vi "Fast Item Remove FuncGlobal.vi"(5 "Action":enum16{"Open or Add", "Close Ref"}(ring), 8 "error in (no error)":errorcluster, 10 "Force Delete (F)":bool, 11 "Item Ref in":T1 format="%.0x") -> (0 "error out":errorcluster, 2 "Deleted?":bool)   [LabVIEW 2011]
doc: "Removes the item and any child items specified by <B>Item Ref in</B>."
uses:
  <vilib>/NI Veristand/Custom Device API/Custom Device Item Ref.ctl
  <vilib>/NI Veristand/Custom Device API/Custom Device API.lvlib
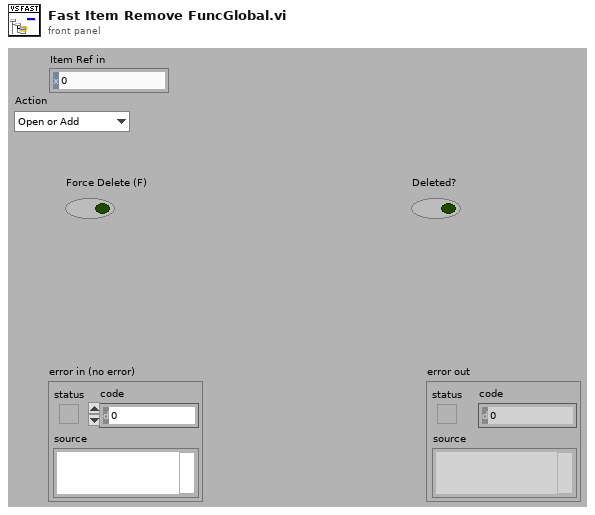
[diagram p1: front panel]
types:
  T1 = typedef "Custom Device API.lvlib/Custom Device Item Ref.ctl" = u64
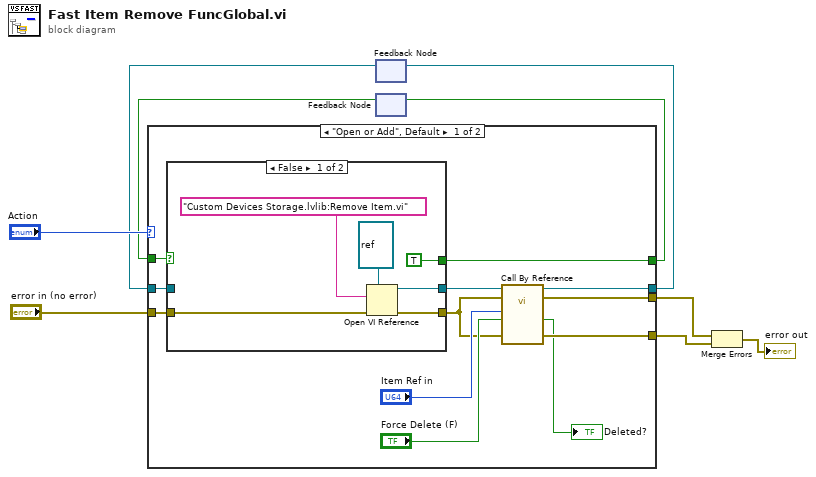
[diagram p0: block diagram]
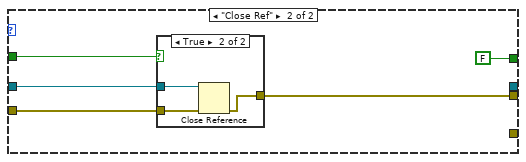
[diagram p3: hidden frame]
diagram:
  n1 = feedback #1() -> (w1:refnum<vi>)  [unwired: 1 in]
  n2 = feedback #2() -> (w4:bool)  [unwired: 1 in]
  n3 = case shown="\"Open or Add\", Default" "Action" {
    tunnel: [w21 _] -> w9
    tunnel: "error in (no error)" -> [w19 w34]
    tunnel: w4 -> [w14 w32]
    tunnel: [w13 FALSE] -> w3
    tunnel: [w12 w31] -> w5
    tunnel: [w11 _] -> w2
    tunnel: w1 -> [w10 w33]
    frame "Open or Add", Default {
      n4 = case shown="False" w14 {
        selector: w14 -> [_ w28]
        tunnel: w19 -> [w25 w29]
        tunnel: [w24 w30] -> w16
        tunnel: [w23 w29] -> w15
        tunnel: [TRUE w28] -> w13
        tunnel: w10 -> [_ w30]
        frame False {
          n5 = Open VI Reference(type specifier VI Refnum (for type only)=refnum<vi> refnum, vi path="Custom Devices Storage.lvlib:Remove Item.vi", error in (no error)=w25) -> (vi reference=w24:refnum<vi>, error out=w23:errorcluster)  [unwired: 3 out]
        }
        frame True {
        }
      }
      n6 = call-by-ref "?"(reference=w16, error in=w15, 8:"error in (no error)"=w15, "Force Delete (F)"="Force Delete (F)", "Item Ref in"="Item Ref in") -> (reference out=w11:refnum<vi>, error out=w12:errorcluster, 0:"error out"=w21:errorcluster, "Deleted?"=→"Deleted?":bool)  [unwired: 7 in]
    }
    frame "Close Ref" {
      n7 = case shown="True" w32 {
        tunnel: w34 -> [w36 w39]
        tunnel: w33 -> [_ w38]
        tunnel: [w36 w37] -> w31
        frame False {
        }
        frame True {
          n8 = Close Reference(reference=w38, error in (no error)=w39) -> (error out=w37:errorcluster)
        }
      }
    }
  }
  n9 = feedback-in #1(w2) -> ()
  n10 = feedback-in #2(w3) -> ()
  n11 = Merge Errors(w5, w9) -> (→"error out":errorcluster)
